vi "Compute DistanceToTarget2.vi"(8 "results":T1, 9 "Camera Type":T3, 11 "Image Src":T2) -> (0 "results out":T1, 3 "Image Dst Out":T2)   [LabVIEW 2019]
doc: "Using the camera lens information and the real world size of the target, use trig and ratios to determine the distance to the target. Also returns the location relative to the image center in a (-1 , 1) coordinate system that may be useful for steering the robot."
uses:
  Camera Types.ctl
  <vilib>/vision/Image Controls.llb/IMAQ Image.ctl
  Target Fields.ctl
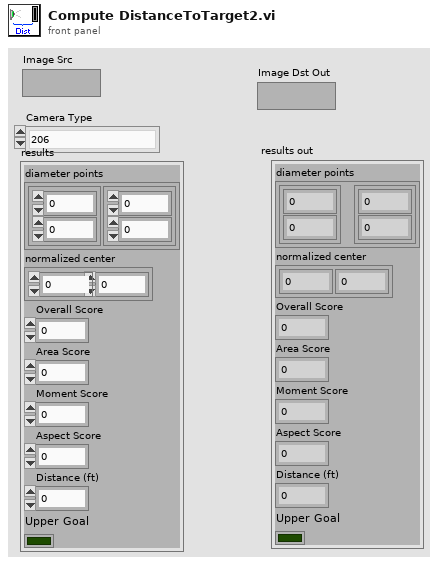
[diagram p1: front panel]
types:
  T1 = typedef "Target Fields.ctl" = cluster{"diameter points":cluster{"first point":cluster{"x":dbl, "y":dbl}, "projected point":cluster{"x":dbl, "y":dbl}}, "normalized center":cluster{"x":dbl, "y":dbl}, "Overall Score":dbl, "Area Score":dbl, "Moment Score":dbl, "Aspect Score":dbl, "Distance (ft)":dbl, "Upper Goal":bool}
  T2 = typedef "IMAQ Image.ctl" = refnum<image>
  T3 = typedef "Camera Types.ctl" = enum16{"206", "1011", "1013", "MS HD3000 square", "MS HD3000 640x480"}
  T4 = cluster{"first point":cluster{"x":dbl, "y":dbl}, "projected point":cluster{"x":dbl, "y":dbl}}
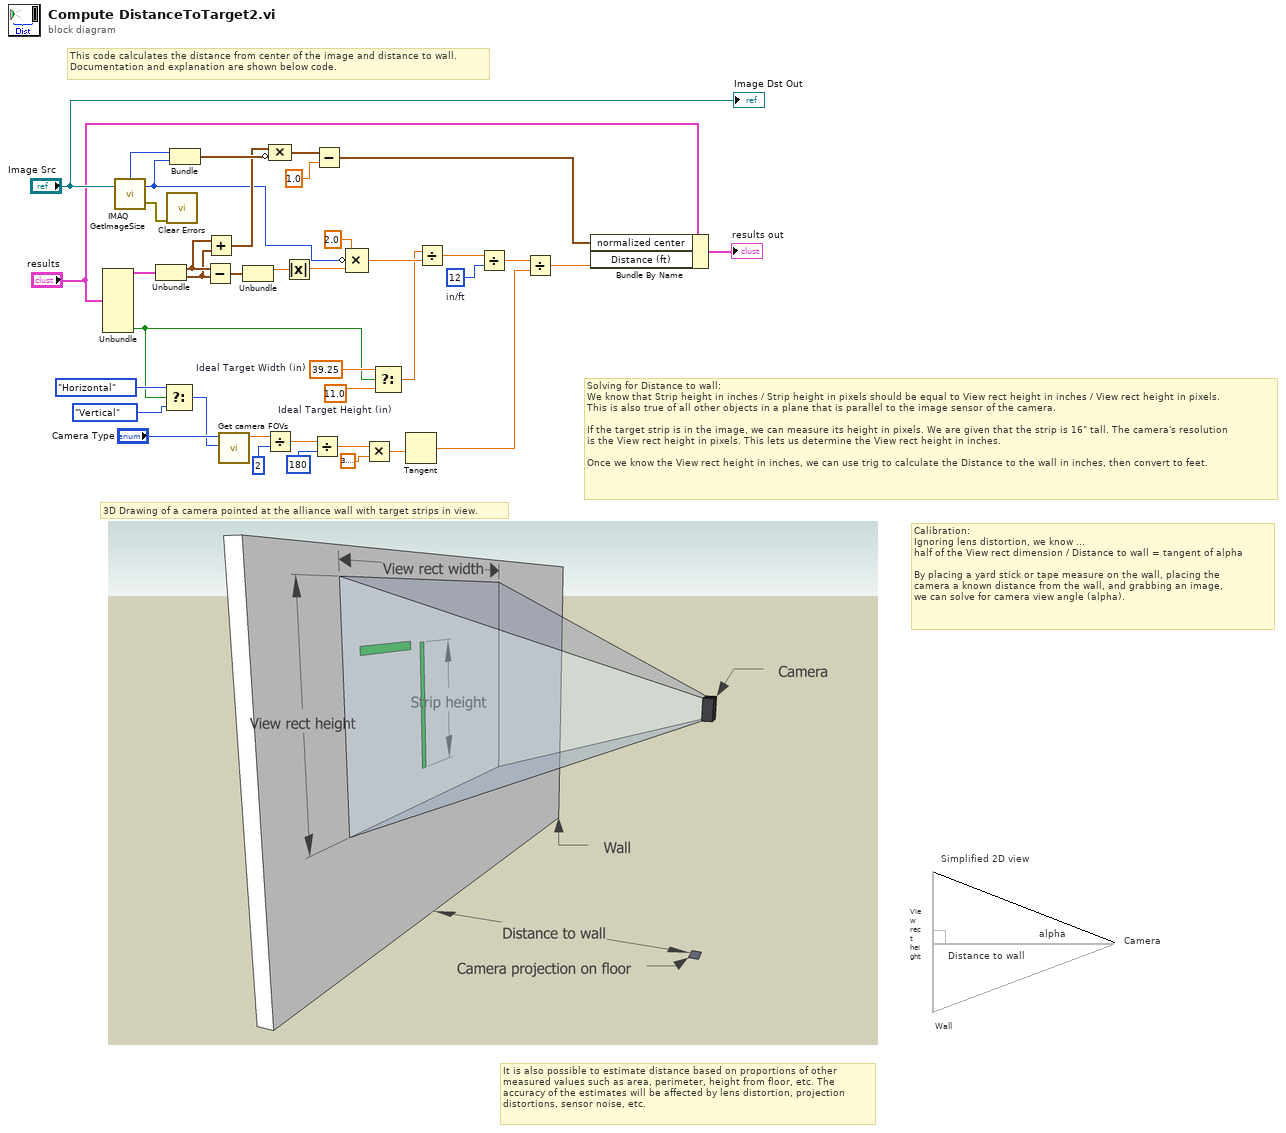
[diagram p0: block diagram]
diagram:
  w6 = 11.0  # Ideal Target Height (in)
  w7 = 39.25  # Ideal Target Width (in)
  w33 = 12  # in/ft
  # "It is also possible to estimate distance based on proportions of other\nmeasured values such as area, perimeter, height from floor, etc. The\naccuracy of the estimates will be affected by lens distortion, projection\ndistortions, sensor noise, etc."
  # "Wall"
  # "Camera"
  # "Simplified 2D view"
  # "Solving for Distance to wall:\nWe know that Strip height in inches / Strip height in pixels should be equal to View rect height in inches / View rect height in pixels.\nThis is also true of all other objects in a plane that is parallel to the image sensor of the camera.\n\nIf the target strip is in the image, we can measure its height in pixels. We are given that the strip is 16\" tall. The camera's resolution\nis the View rect height in pixels. This lets us determine the View rect height in inches.\n\nOnce we know the View rect height in inches, we can use trig to calculate the Distance to the wall in inches, then convert to feet."
  # "3D Drawing of a camera pointed at the alliance wall with target strips in view."
  # "Distance to wall"
  # "View rect height"
  # "alpha"
  # "Calibration:\nIgnoring lens distortion, we know ...\nhalf of the View rect dimension / Distance to wall = tangent of alpha\n\nBy placing a yard stick or tape measure on the wall, placing the\ncamera a known distance from the wall, and grabbing an image,\nwe can solve for camera view angle (alpha)."
  # "This code calculates the distance from center of the image and distance to wall.\nDocumentation and explanation are shown below code."
  n1 = Unbundle("results") -> ("diameter points"=w16:T4, "Upper Goal"=w1:bool)  [unwired: 6 out]
  n2 = call "IMAQ GetImageSize"("Image"="Image Src") -> ("Y Resolution"=w8:i32, "X Resolution"=w17:i32, "error out"=w26:errorcluster)  [unwired: 3 in]
  n3 = Unbundle(w16) -> ("first point"=w12:cluster{"x":dbl, "y":dbl}, "projected point"=w11:cluster{"x":dbl, "y":dbl})
  n4 = Select(t=enum16{"Horizontal", "Vertical", "Diagonal"}."Horizontal" ("Angle"), s=w1, f=enum16{"Horizontal", "Vertical", "Diagonal"}."Vertical" ("Angle")) -> (s? t:f=w3:enum16{"Horizontal", "Vertical", "Diagonal"})
  n5 = call <vilib>:"Clear Errors.vi"("error in (no error)"=w26) -> ()  [unwired: 5 in, 2 out]
  n6 = Bundle("X Resolution"=w17, "Y Resolution"=w8) -> (w13:cluster{"X Resolution":i32, "Y Resolution":i32})  [unwired: 1 in]
  n7 = Subtract(x=w12, y=w11) -> (x-y=w22:cluster{"x":dbl, "y":dbl})
  n8 = Add(x=w12, y=w11) -> (x+y=w10:cluster{"x":dbl, "y":dbl})
  n9 = call "Get camera FOVs.vi"("Type"=w3, "Camera Type"="Camera Type") -> ("FOV"=w30:dbl)  [unwired: 8 in, 1 out]
  n10 = Unbundle(w22) -> ("x"=w21:dbl)  [unwired: 1 out]
  n11 = Divide(x=w30, y=2) -> (x/y=w36:dbl)
  n12 = Compound Arithmetic op=MULTIPLY(w10, invert w13) -> (w15:cluster{dbl, dbl})
  n13 = Absolute Value(x=w21) -> (abs(x)=w23:dbl)
  n14 = Divide(x=w36, y=180) -> (x/y=w35:dbl)
  n15 = Subtract(x=w15, y=1.0) -> (x-y=w14:cluster{dbl, dbl})
  n16 = Compound Arithmetic op=MULTIPLY(2.0, invert w8, w23) -> (w27:dbl)
  n17 = Multiply(x=w35, y=3.141592653589793) -> (x*y=w37:dbl)
  n18 = Select(t=w7, s=w1, f=w6) -> (s? t:f=w5:dbl)
  n19 = Tangent(1:w37) -> (0:w32:dbl)
  n20 = Divide(x=w5, y=w27) -> (x/y=w24:dbl)
  n21 = Divide(x=w24, y=w33) -> (x/y=w31:dbl)
  n22 = Divide(x=w31, y=w32) -> (x/y=w18:dbl)
  n23 = Bundle By Name(cluster="results", "normalized center"=w14, "Distance (ft)"=w18) -> (→"results out":T1)
  "Image Dst Out" <- "Image Src"
